vi "Read Input Registers.vi"(8 "error in":errorcluster, 9 "number of inputs":u16, 10 "starting address":u16, 11 "Modbus master in":refnum<class "Modbus Master.lvclass">) -> (0 "error out":errorcluster, 2 "register values":u16[](array[numeric]), 3 "Modbus master out":refnum<class "Modbus Master.lvclass">)   [LabVIEW 2014, in "MyLib.lvlib" / "Modbus Master.lvclass"]
doc: "Reads <B>number of inputs</B> input registers starting at <B>starting address</B> from the device."
uses:
  Modbus Master.lvclass
  Modbus Master.lvclass/Modbus Master.ctl
  Modbus API.lvclass/Modbus API.ctl
  Transmission Data Unit/Transmission Data Unit.lvclass
  Modbus API.lvclass
  Master Function Definition/Master Function Definition.lvclass
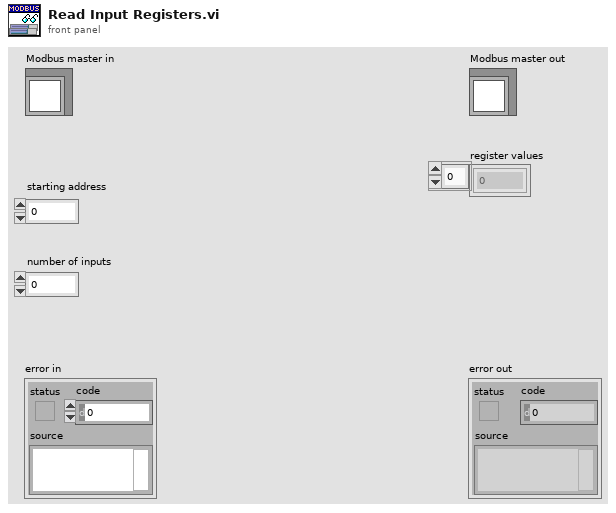
[diagram p1: front panel]
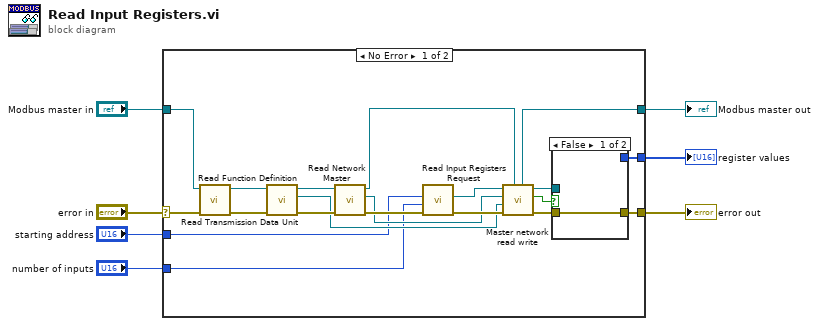
[diagram p0: block diagram]
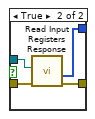
[diagram p2: hidden frame]
diagram:
  n1 = case shown="No Error" "error in" {
    selector: "error in" -> [w18 w34]
    tunnel: [w19 w34] -> w6
    tunnel: [w12 w33] -> w5
    tunnel: "Modbus master in" -> [w11 w33]
    tunnel: [w13 _] -> w3
    tunnel: "starting address" -> [w10 _]
    tunnel: "number of inputs" -> [w9 _]
    frame No Error {
      n2 = call "Read Function Definition.vi"("error in"=w18, "Modbus master in"=w11) -> ("error out"=w25:errorcluster, "Modbus master out"=w26:refnum<class "Modbus Master.lvclass">)  [unwired: 7 in, 1 out]
      n3 = call "Read Transmission Data Unit.vi"("error in"=w25, "Modbus instance in"=w26) -> ("error out"=w27:errorcluster, "transmission data unit"=w14:refnum<class "Transmission Data Unit.lvclass">, "Modbus instance out"=w24:refnum<class "Modbus Master.lvclass">)  [unwired: 7 in]
      n4 = call "Read Network Master.vi"("error in"=w27, "Modbus master in"=w24) -> ("error out"=w20:errorcluster, "network master"=w15:refnum<class "Network Master.lvclass">, "Modbus master out"=w21:refnum<class "Modbus Master.lvclass">)  [unwired: 7 in]
      n5 = call "Read Input Registers Request.vi"("error in"=w20, "Number of Registers"=w9, "Starting Address"=w10) -> ("error out"=w22:errorcluster, "modbus data unit out"=w16:refnum<class "Modbus Data Unit.lvclass">)  [unwired: 7 in]
      n6 = call "Master network read write.vi"("Modbus master in"=w21, "error in"=w22, "transmission data unit in"=w14, "network master in"=w15, "Modbus data unit in"=w16) -> ("error out"=w23:errorcluster, "PDU Valid?"=w8:bool, "Modbus data unit out"=w17:refnum<class "Modbus Data Unit.lvclass">, "Modbus master out"=w12:refnum<class "Modbus Master.lvclass">)  [unwired: 3 in]
      n7 = case shown="False" w8 {
        tunnel: w23 -> [w28 w32]
        tunnel: [w28 w31] -> w19
        tunnel: w17 -> [_ w30]
        tunnel: [_ w29] -> w13
        frame False {
        }
        frame True {
          n8 = call "Read Input Registers Response.vi"("error in"=w32, "modbus data unit in"=w30) -> ("error out"=w31:errorcluster, "Register Values"=w29:u16[])  [unwired: 7 in, 1 out]
        }
      }
    }
    frame Error {
    }
  }
  "error out" <- w6
  "Modbus master out" <- w5
  "register values" <- w3
